vi "Monitor Ques.vi"() -> ()   [LabVIEW 2025]
panel:
  in  "stop":bool
  out "# pending remove 2":i32
  out "# pending insert 2":i32
  out "# pending insert":i32
  out "# pending remove":i32
  in  "serial channels":string[](array[string])=["SI0", "SI1"]
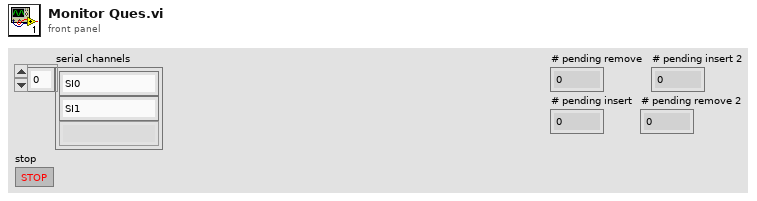
[diagram p1: front panel]
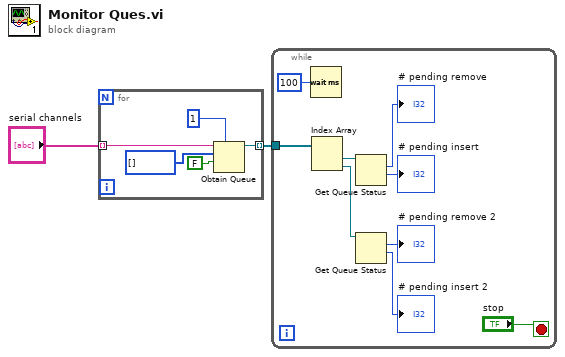
[diagram p0: block diagram]
diagram:
  n1 = for {
    tunnel: "serial channels" -> [w7] mode=indexing
    tunnel: [w5] -> w1 mode=indexing
    n2 = Obtain Queue(max queue size (-1, unlimited)=1, name (unnamed)=w7, element data type=u32[] [] ("Image Pixels (U32)"), create if not found? (T)=FALSE) -> (queue out=w5:refnum<queue>)  [unwired: 1 in, 2 out]
  }
  n3 = while {
    tunnel: w1 -> [w16]
    stop <- "stop" stop-if-true
    n4 = Wait (ms)(milliseconds to wait=u32 100) -> ()  [unwired: 1 out]
    n5 = Index Array(array=w16) -> (element #1=w15:refnum<queue>, element #2=w10:refnum<queue>)  [unwired: 2 in]
    n6 = Get Queue Status(queue=w15) -> (# pending remove=→"# pending remove":i32, # pending insert=→"# pending insert":i32)  [unwired: 2 in, 6 out]
    n7 = Get Queue Status(queue=w10) -> (# pending remove=→"# pending remove 2":i32, # pending insert=→"# pending insert 2":i32)  [unwired: 2 in, 6 out]
  }
